vi "XIPIN_AXI_EPC_2_0.vi"   [LabVIEW 2017]
doc: "This specification defines the architecture and interface requirements for the External Peripheral Controller (AXI EPC IP Core).\n------------------------------------\n<b>Need License</b> : No\n<b>Interface</b> : AXI4"
uses:
  <vilib>/rvi/XilinxIP/XIPIN_XNode/niFpgaXIPIN.xnode
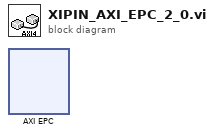
[diagram p0: block diagram]
diagram:
  n1 = xnode ("AXI EPC")() -> ()
